vi "Shutdown.vi"(8 "error in":errorcluster, 11 "device data model in":refnum<class "Standard Data Model.lvclass">) -> (0 "error out":errorcluster)   [LabVIEW 2013, in "Modbus Library - Advance.lvlib" / "Standard Data Model.lvclass"]
doc: "This VI is responsible for deleting the device data model."
uses:
  Standard Data Model.lvclass
  Standard Data Model.lvclass/Standard Data Model.ctl
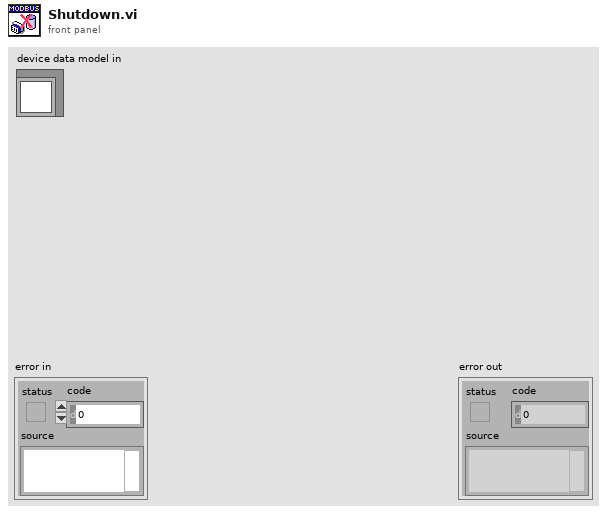
[diagram p1: front panel]
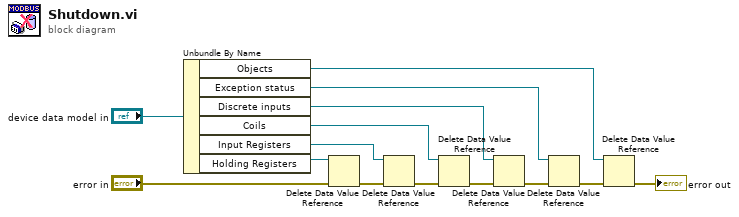
[diagram p0: block diagram]
diagram:
  n1 = Unbundle By Name("device data model in") -> ("Objects"=w2:refnum<data-value>, "Exception status"=w1:refnum<data-value>, "Discrete inputs"=w13:refnum<data-value>, "Coils"=w12:refnum<data-value>, "Input Registers"=w11:refnum<data-value>, "Holding Registers"=w10:refnum<data-value>)
  n2 = Delete Data Value Reference(data value reference=w10, error in="error in") -> (error out=w9:errorcluster)  [unwired: 1 out]
  n3 = Delete Data Value Reference(data value reference=w11, error in=w9) -> (error out=w8:errorcluster)  [unwired: 1 out]
  n4 = Delete Data Value Reference(data value reference=w12, error in=w8) -> (error out=w7:errorcluster)  [unwired: 1 out]
  n5 = Delete Data Value Reference(data value reference=w13, error in=w7) -> (error out=w3:errorcluster)  [unwired: 1 out]
  n6 = Delete Data Value Reference(data value reference=w1, error in=w3) -> (error out=w5:errorcluster)  [unwired: 1 out]
  n7 = Delete Data Value Reference(data value reference=w2, error in=w5) -> (error out=→"error out":errorcluster)  [unwired: 1 out]
